vi "Tecella_FETAnalyser.vi"() -> ()   [LabVIEW 2009]
doc: "FET Analysis Code\n(C) Michael Walker 2014\nFree to re use and distribute for non commercial use. All rights reserved for commercial use.\nRed dsitrbution and modification must keep this license intact.\nSoftware is provided as is. The author accepts no responsibility for loss arising out of use of this program."
uses:
  TecellaChannel/TecellaChannel.lvclass
  <vilib>/measure/madcrms.llb/Basic Averaged DC-RMS for 1 Chan.vi
  TecellaClient/TecellaClient.lvclass
  <vilib>/measure/NI_MAPro.lvlib
panel:
  out "Running?":bool
  out "Igs nA":dbl format="%0.2e"
  in  "Channel 2":i8=2
  in  "Channel":i8
  out "Gate Resistance":dbl=-654868.3548789481 format="%#.4e"
  out "Gate IV":cluster{"Y":dbl[], "Y":dbl[]}[](graph)=[{"Y"=[90.50541857309688, 90.84377717312921, 91.26591980808492, 91.21758286507902, 91.67162788253441, 91.97325040553291], "Y"=[-1.1330458045852234e-05, -1.131434573173331e-05, -1.1781602836448501e-05, -1.2158630983030932e-05, -1.2596885922907083e-05, -1.1881499183117178e-05]}, {"Y"=[90.50541857309688, 90.84377717312921, 91.26591980808492, 91.21758286507902, 91.67162788253441, 91.97325040553291], "Y"=[-1.1358748353855137e-05, -1.1580328693617457e-05, -1.1856776546495164e-05, -1.1825122212149017e-05, -1.2122461925771009e-05, -1.2319984971201474e-05]}]
  in  "Recording?":bool
  in  "Dtitles":string[](array[string])
  in  "Clear Data":bool
  out "Data":cluster{"Y":dbl[], "Y":dbl[]}[](graph)
  out "Igs versus Vds":cluster{"Y":dbl[], "Y":dbl[]}[](graph)=[{"Y"=[90.50541857309688, 90.84377717312921, 91.26591980808492, 91.21758286507902, 91.67162788253441, 91.97325040553291], "Y"=[-1.1330458045852234e-05, -1.131434573173331e-05, -1.1781602836448501e-05, -1.2158630983030932e-05, -1.2596885922907083e-05, -1.1881499183117178e-05]}, {"Y"=[90.50541857309688, 90.84377717312921, 91.26591980808492, 91.21758286507902, 91.67162788253441, 91.97325040553291], "Y"=[-1.1358748353855137e-05, -1.1580328693617457e-05, -1.1856776546495164e-05, -1.1825122212149017e-05, -1.2122461925771009e-05, -1.2319984971201474e-05]}]
  out "Vgs FileNo":dbl
  out "Ids/Vds No":dbl
  out "File Path for saving":path=path "D:/Data/101116/101116_1/101116_1_FET0_100Hz_"
  in  "Details":string
  in  "Folder Path":path=path "D:/Data"
  out "File No":dbl
  out "Saving Data":bool
  out "File Name Out":path
  out "Vds Progress":u8(slide) scale=0.0..100.0
  out "Vgs Progress":u8(slide) scale=0.0..100.0
  in  "Start/Stop Recording":bool
  in  "Record All Data":bool
  in  "Vds Stabilisation":u32=700
  in  "Vgs Stabilisation":u32=600
  in  "clear":bool
  out "Channel Conducitivty (uS)":dbl format="%0.3e"
  out "Channel Resistance":dbl format="%#_3e"
  out "Live Channel Resistance":dbl format="%#_3e"
  out "Live channel Conductivity uS":dbl format="%#_3e"
  out "Vgs mV":dbl format="%0.2p"
  in  "Sample Freq Hz":dbl=100.0
  out "Vds mV":dbl format="%0.2p"
  in  "Set Vds mV":dbl
  in  "Set Vgs mV":dbl
  in  "stop":bool
  out "Ids nA":dbl format="%0.2e"
  in  "Samples to read":dbl=1024.0
  out "Measured Igs":dbl[][](graph)
  out "Masured Ids":dbl[][](graph)
  in  "Measure Channel Conductivity":bool
  in  "With Vds Sweep":bool
  in  "NoSteps":dbl=10.0
  in  "No steps":dbl=10.0
  in  "Vgs Min":dbl=-100.0
  in  "Vgs Max":dbl=100.0
  in  "Vds Min":dbl=-100.0
  in  "Vds Max":dbl=100.0
  in  "FET Analyse":bool
  out "S against Vds":cluster{"Y":dbl[], "Y":dbl[]}[](graph)
  out "Ids Agsint Vds":cluster{"Y":dbl[], "Y":dbl[]}[](graph)
  # "Note currents are recorded consecutivly and sample \nrate is incorrect"
  # "Drain Source Voltage Sweep"
  # "Gate Source Voltage Sweep"
  # "NB new file created each time recording is started"
  # "Controls actual recording"
  # "Used to indicate if the current file has been recorded into"
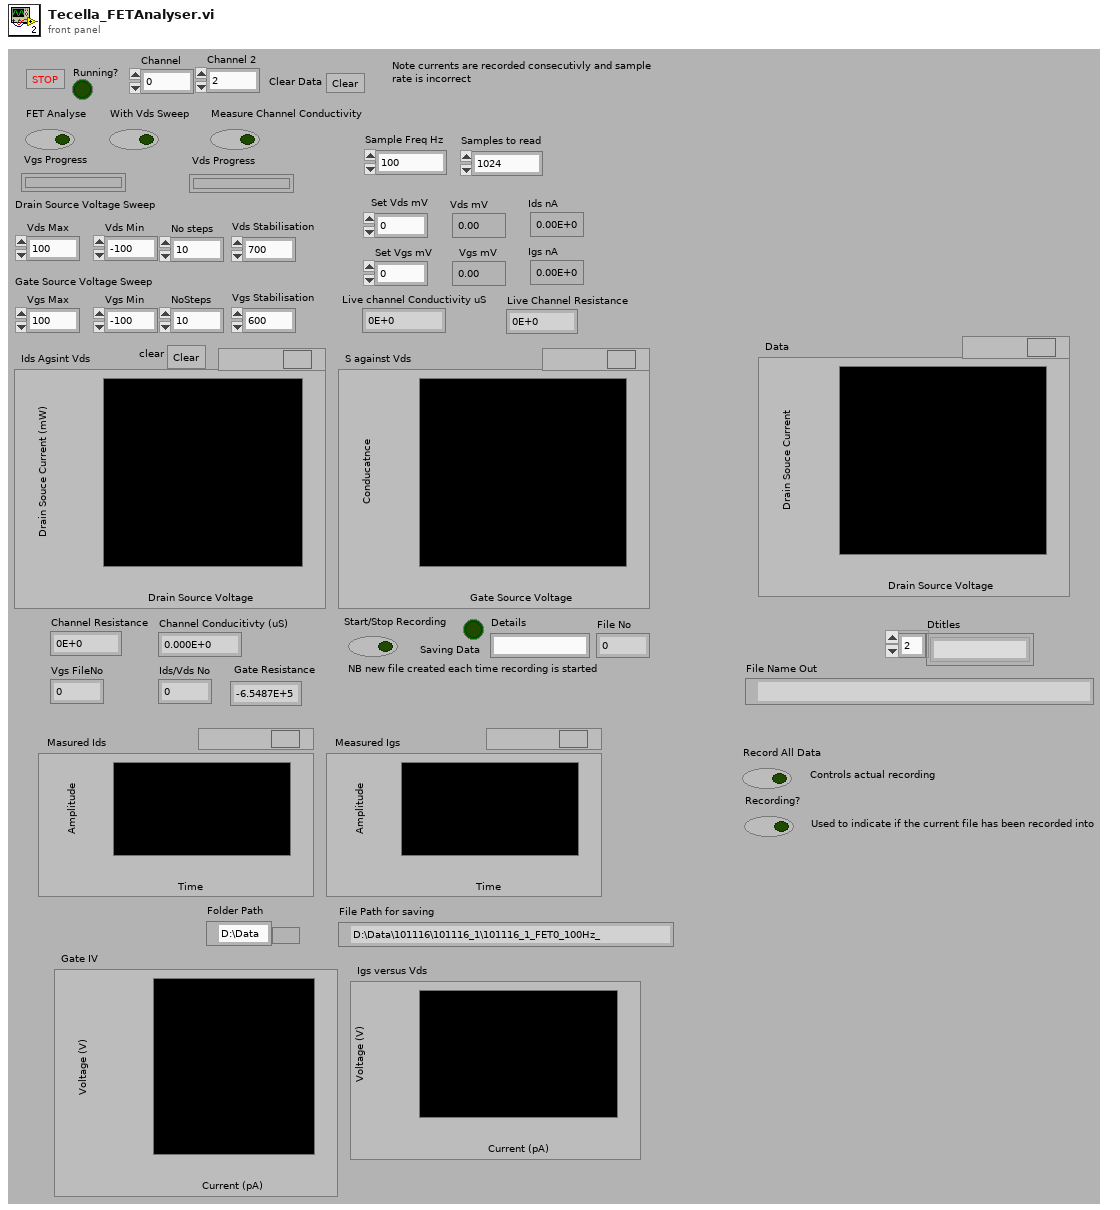
[diagram p1: front panel]
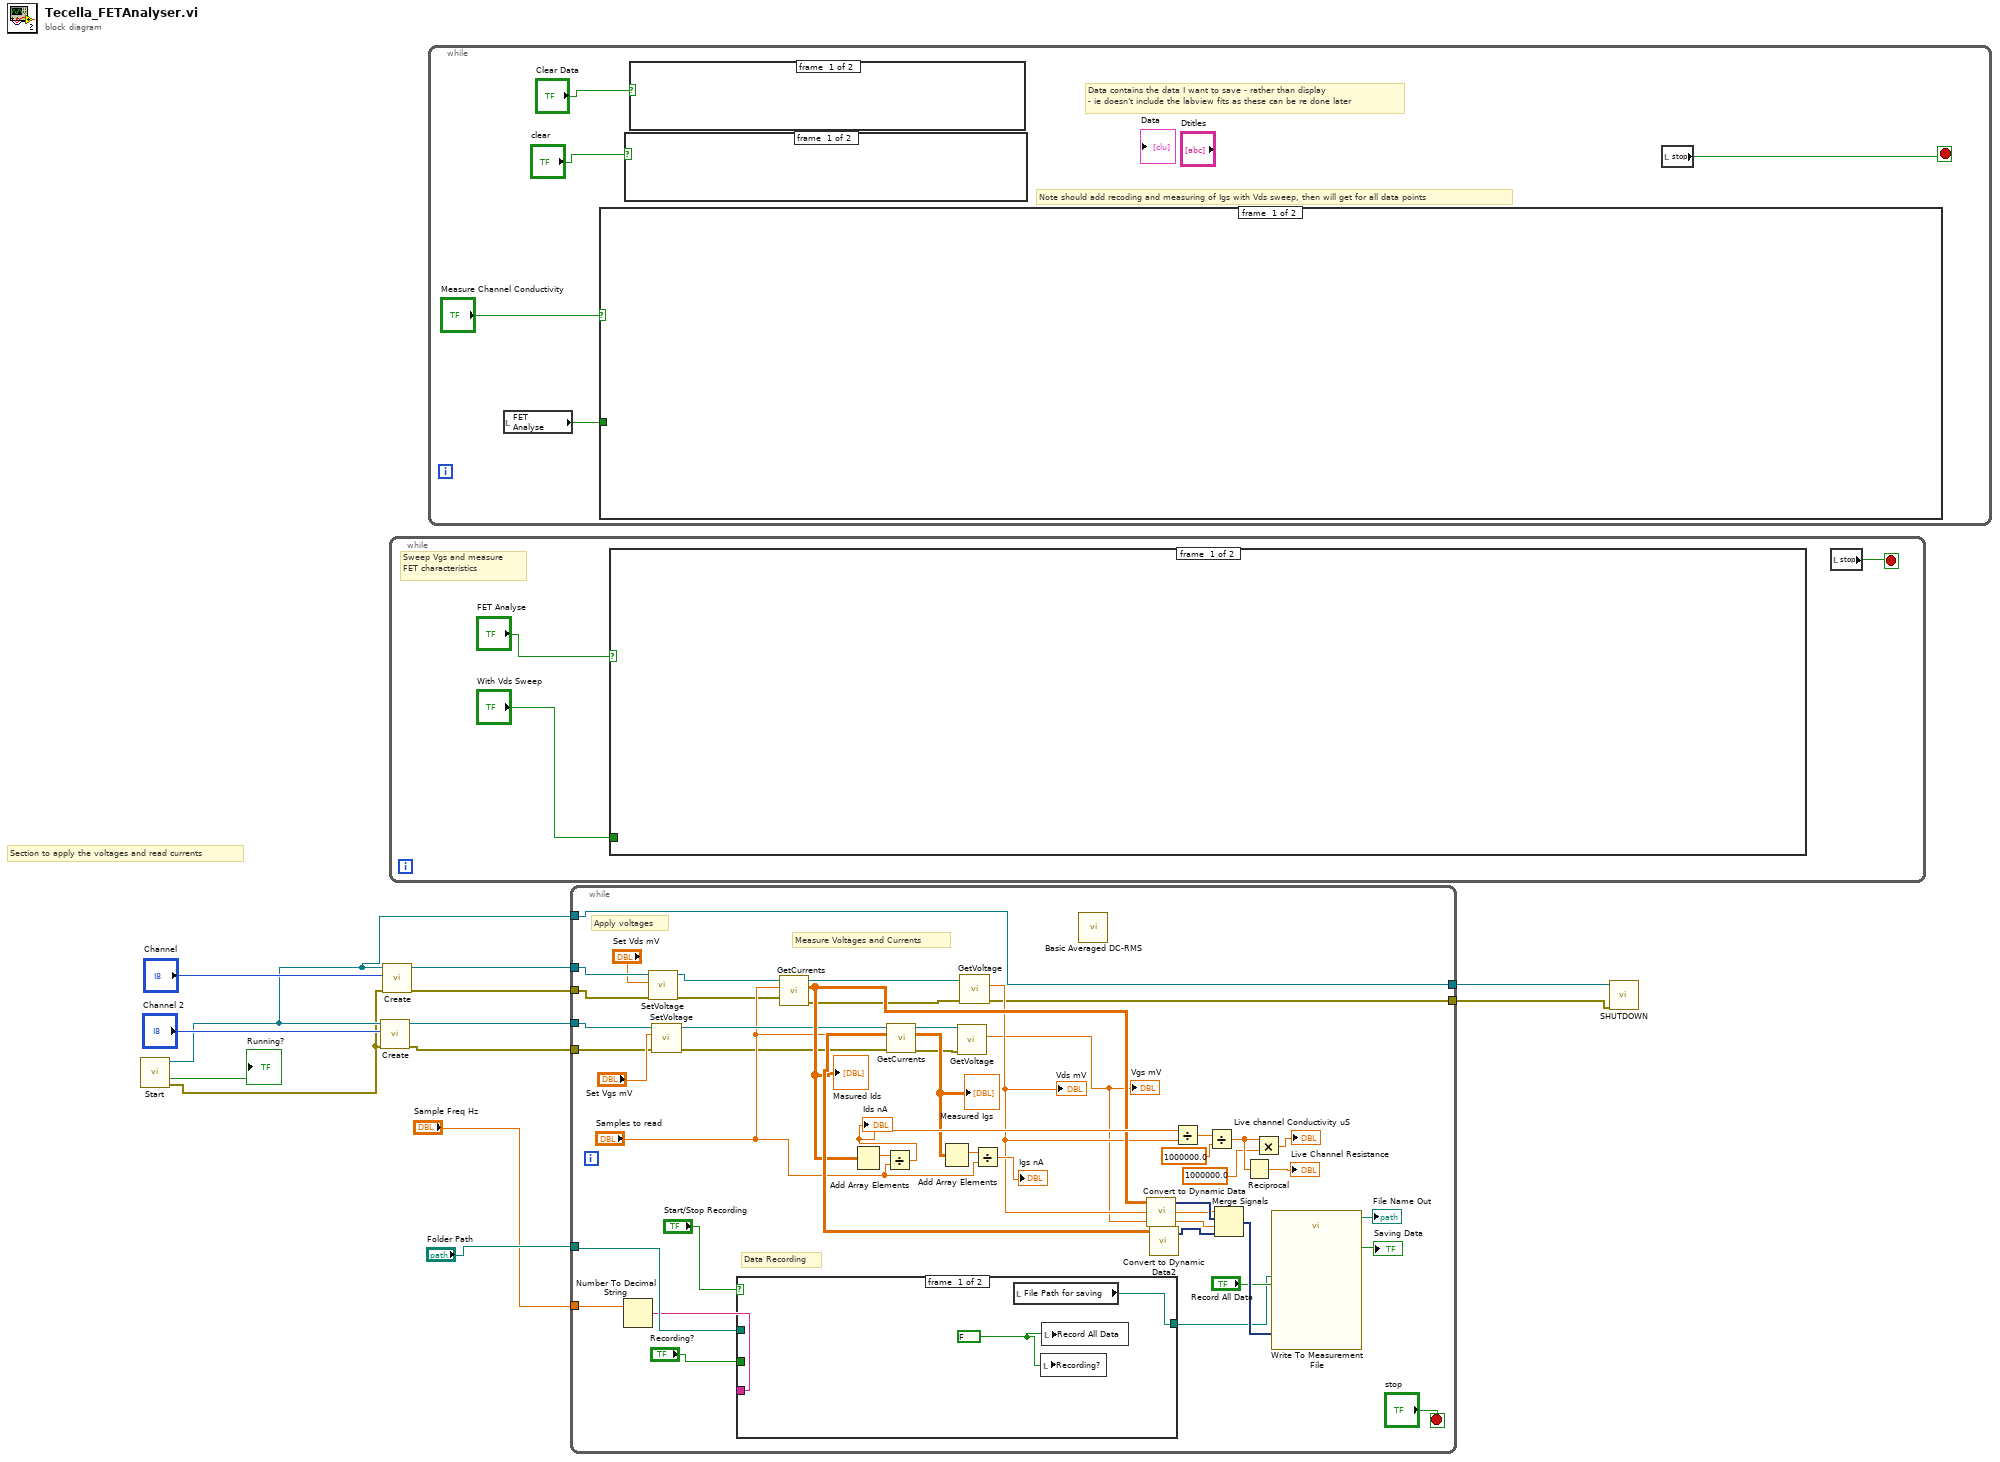
[diagram p0: block diagram]
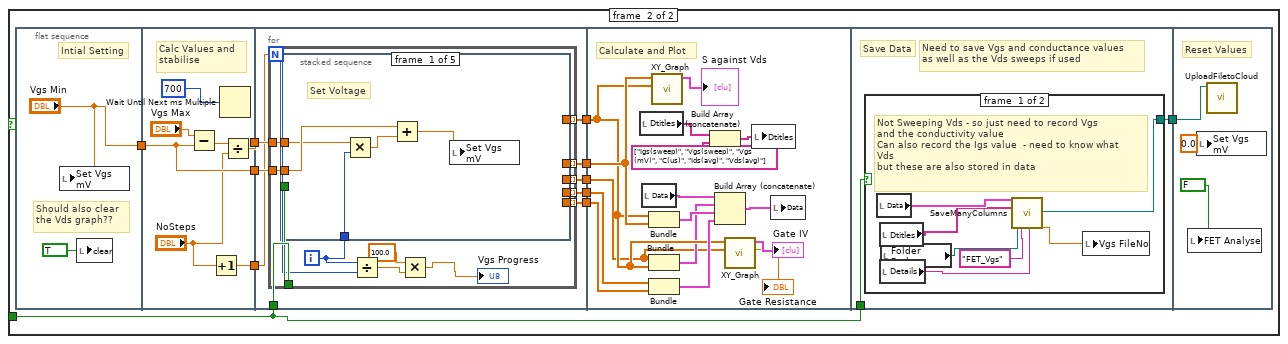
[diagram p2: hidden frame]
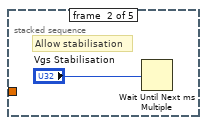
[diagram p3: hidden frame]
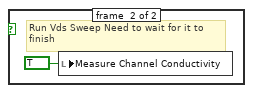
[diagram p5: hidden frame]
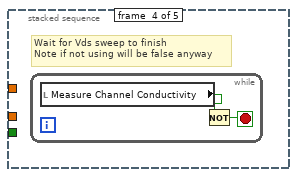
[diagram p6: hidden frame]
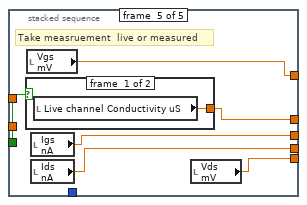
[diagram p7: hidden frame]
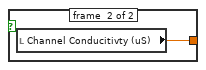
[diagram p8: hidden frame]
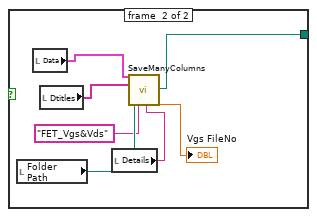
[diagram p9: hidden frame]
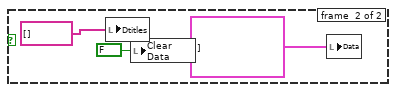
[diagram p10: hidden frame]
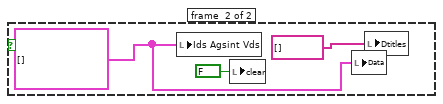
[diagram p11: hidden frame]
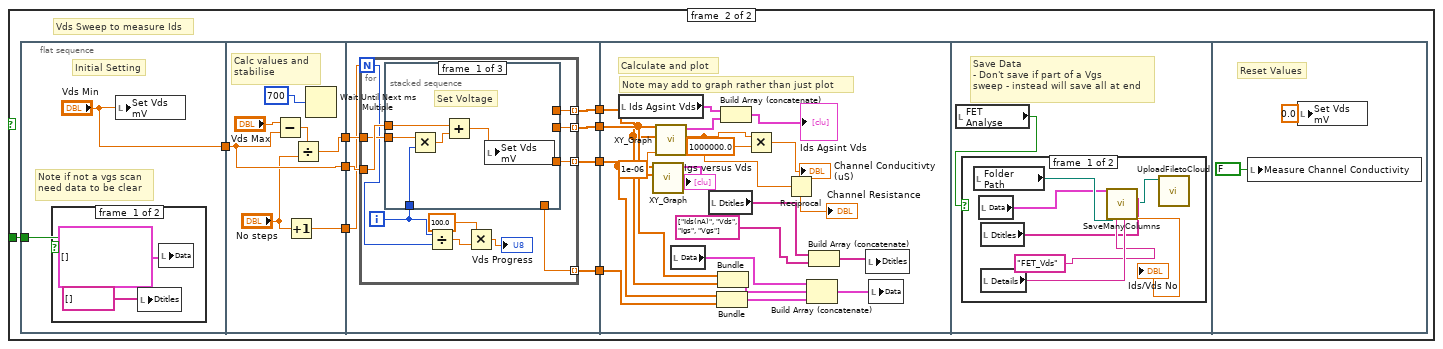
[diagram p12: hidden frame]
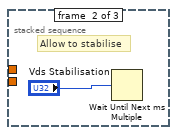
[diagram p14: hidden frame]
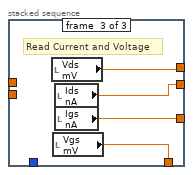
[diagram p15: hidden frame]
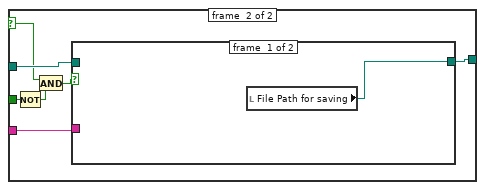
[diagram p17: hidden frame]
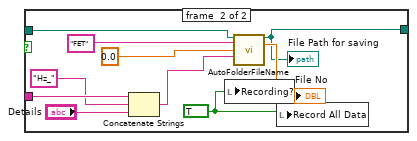
[diagram p18: hidden frame]
diagram:
  # "Section to apply the voltages and read currents"
  n1 = call "Start.vi"() -> ("TecellaClient"=w6:refnum<class "TecellaClient.lvclass">, "Running?"=→"Running?":bool, "error out"=w1:errorcluster)  [unwired: 11 in, 2 out]
  n2 = call "Create.vi"("error in (no error)"=w1, "Channel"="Channel 2", "TecellaClient.lvclass"=w6) -> ("error out"=w2:errorcluster, "TecellaChannel out"=w7:refnum<class "TecellaChannel.lvclass">)  [unwired: 7 in]
  n3 = call "Create.vi"("error in (no error)"=w1, "Channel"="Channel", "TecellaClient.lvclass"=w6) -> ("error out"=w3:errorcluster, "TecellaChannel out"=w8:refnum<class "TecellaChannel.lvclass">)  [unwired: 7 in]
  n4 = while {
    stop <- w14 stop-if-true
    # "Sweep Vgs and measure \nFET characteristics"
    n5 = case shown="True" "FET Analyse" {
      tunnel: "With Vds Sweep" -> [_ w22]
      frame #0 {
      }
      frame #1 {
        n6 = flat-sequence {
          tunnel: ["Vgs Min"] -> w27
          tunnel: w27 -> [w33]
          tunnel: [w33] -> w24
          tunnel: [w32] -> w23
          tunnel: [w30] -> w18
          tunnel: w22 -> [w45]
          tunnel: [w44] -> w26
          tunnel: [w43] -> w25
          tunnel: w24 -> [w42]
          tunnel: w23 -> [w41]
          tunnel: [w40] -> w21
          tunnel: [w39] -> w20
          tunnel: [w38] -> w19
          tunnel: w18 -> [w37]
          tunnel: w26 -> [w80]
          tunnel: w25 -> [w87]
          tunnel: w21 -> [w77]
          tunnel: w20 -> [w85]
          tunnel: w19 -> [w86]
          tunnel: w22 -> [w94]
          tunnel: [w93] -> w17
          tunnel: w17 -> [w109]
          frame #0 {
            # "Should also clear \nthe Vds graph??"
            # "Intial Setting"
            n7 = local write "Set Vgs mV"("Vgs Min") -> ()
            n8 = local write "clear"(TRUE ("clear")) -> ()
          }
          frame #1 {
            # "Calc Values and \nstabilise"
            n9 = Subtract(x="Vgs Max", y=w33) -> (x-y=w36:dbl)
            n10 = Increment(x="NoSteps") -> (x+1=w30:dbl)
            n11 = Wait Until Next ms Multiple(millisecond multiple=u32 700) -> ()  [unwired: 1 out]
            n12 = Divide(x=w36, y="NoSteps") -> (x/y=w32:dbl)
          }
          frame #2 {
            n13 = for {
              N: w37 -> [w53]
              tunnel: w45 -> [w58]
              tunnel: [w57] -> w44 mode=indexing
              tunnel: [w56] -> w43 mode=indexing
              tunnel: w42 -> [w55]
              tunnel: w41 -> [w52]
              tunnel: [w48] -> w40 mode=indexing
              tunnel: [w47] -> w39 mode=indexing
              tunnel: [w46] -> w38 mode=indexing
              i -> [w54]
              n14 = stacked-sequence {
                tunnel: w58 -> [_ _ w65 _ w74]
                tunnel: [_ _ _ _ w73] -> w57
                tunnel: [_ _ _ _ w72] -> w56
                tunnel: w54 -> [w63 _ _ _ _]
                tunnel: w55 -> [w61 _ _ _ _]
                tunnel: w52 -> [w59 _ _ _ _]
                tunnel: [_ _ _ _ w69] -> w48
                tunnel: [_ _ _ _ w71] -> w47
                tunnel: [_ _ _ _ w70] -> w46
                frame #0 {
                  # "Set Voltage"
                  n15 = Multiply(x=w59, y=w63) -> (x*y=w62:dbl)
                  n16 = Add(x=w61, y=w62) -> (x+y=w60:dbl)
                  n17 = local write "Set Vgs mV"(w60) -> ()
                }
                frame #1 {
                  # "Allow stabilisation"
                  n18 = Wait Until Next ms Multiple(millisecond multiple="Vgs Stabilisation") -> ()  [unwired: 1 out]
                }
                frame #2 {
                  # "Now run Vds sweep and wait for it to finish\nOr just take the live values"
                  n19 = case shown="True" w65 {
                    frame #0 {
                      # "Just take the live values"
                    }
                    frame #1 {
                      # "Run Vds Sweep Need to wait for it to \nfinish"
                      n20 = local write "Measure Channel Conductivity"(TRUE ("Measure Channel Conductivity")) -> ()
                    }
                  }
                }
                frame #3 {
                  # "Wait for Vds sweep to finish\nNote if not using will be false anyway"
                  n21 = while {
                    stop <- w68 stop-if-true
                    n22 = local read "Measure Channel Conductivity"() -> (w67:bool)
                    n23 = Not(x=w67) -> (.not. x?=w68:bool)
                  }
                }
                frame #4 {
                  # "Take measruement  live or measured"
                  n24 = case shown="True" w74 {
                    tunnel: [w75 w76] -> w72
                    frame #0 {
                      n25 = local read "Live channel Conductivity uS"() -> (w75:dbl)
                    }
                    frame #1 {
                      n26 = local read "Channel Conducitivty (uS)"() -> (w76:dbl)
                    }
                  }
                  n27 = local read "Vgs mV"() -> (w73:dbl)
                  n28 = local read "Igs nA"() -> (w69:dbl)
                  n29 = local read "Ids nA"() -> (w70:dbl)
                  n30 = local read "Vds mV"() -> (w71:dbl)
                }
              }
              n31 = Divide(x=w54, y=w53) -> (x/y=w50:dbl)
              n32 = Multiply(x=100.0, y=w50) -> (x*y=→"Vgs Progress":dbl)
            }
          }
          frame #3 {
            # "Calculate and Plot"
            n33 = local read "Dtitles"() -> (w90:string[])
            n34 = local read "Data"() -> (w79:cluster{"Y":dbl[], "Y":dbl[]}[])
            n35 = Bundle(w80, w87) -> (w81:cluster{dbl[], dbl[]})  [unwired: 1 out]
            n36 = Bundle(w77, w80) -> (w78:cluster{dbl[], dbl[]})  [unwired: 1 out]
            n37 = Bundle(w86, w85) -> (w82:cluster{dbl[], dbl[]})  [unwired: 1 out]
            n38 = call "XY_Graph.vi"("X"=w80, "Y"=w87) -> ("I-V Curve"=→"S against Vds":cluster{"Y":dbl[], "Y":dbl[]}[])  [unwired: 8 in, 1 out]
            n39 = Build Array (concatenate)(w90, string[] ["Igs(sweep)", "Vgs(sweep)", "Vgs (mV)", "C(us)", "Ids(avg)", "Vds(avg)"] ("ColumnTitle Array")) -> (w89:string[])
            n40 = Build Array (concatenate)(w79, w78, w81, w82) -> (w91:cluster{"Y":dbl[], "Y":dbl[]}[])
            n41 = call "XY_Graph.vi"("X"=w77, "Y"=w80) -> ("Gradient"=→"Gate Resistance":dbl, "I-V Curve"=→"Gate IV":cluster{"Y":dbl[], "Y":dbl[]}[])  [unwired: 8 in]
            n42 = local write "Dtitles"(w89) -> ()
            n43 = local write "Data"(w91) -> ()
          }
          frame #4 {
            # "Need to save Vgs and conductance values\nas well as the Vds sweeps if used"
            # "Save Data"
            n44 = case shown="False" w94 {
              tunnel: [w95 w102] -> w93
              frame #0 {
                # "Not Sweeping Vds - so just need to record Vgs\nand the conductivity value \nCan also record the Igs value  - need to know what \nVds\nbut these are also stored in data"
                n45 = local read "Data"() -> (w100:cluster{"Y":dbl[], "Y":dbl[]}[])
                n46 = local read "Dtitles"() -> (w96:string[])
                n47 = local read "Details"() -> (w97:string)
                n48 = local read "Folder Path"() -> (w101:path)
                n49 = call "SaveManyColumns.vi"("InputCluster"=w100, "ColumnTitle Array"=w96, "Folder Path"=w101, "Capillary Type"="FET_Vgs" ("Comments"), "Details"=w97) -> ("Saved Path"=w95:path, "File No"=w99:dbl)  [unwired: 20 in, 1 out]
                n50 = local write "Vgs FileNo"(w99) -> ()
              }
              frame #1 {
                n51 = local read "Folder Path"() -> (w107:path)
                n52 = local read "Data"() -> (w104:cluster{"Y":dbl[], "Y":dbl[]}[])
                n53 = local read "Dtitles"() -> (w103:string[])
                n54 = local read "Details"() -> (w105:string)
                n55 = call "SaveManyColumns.vi"("InputCluster"=w104, "ColumnTitle Array"=w103, "Folder Path"=w107, "Capillary Type"="FET_Vgs&Vds" ("Comments"), "Details"=w105) -> ("Saved Path"=w102:path, "File No"=→"Vgs FileNo":dbl)  [unwired: 20 in, 1 out]
              }
            }
          }
          frame #5 {
            # "Reset Values"
            n56 = local write "FET Analyse"(FALSE ("FET Analyse")) -> ()
            n57 = local write "Set Vgs mV"(0.0 ("Set Vgs")) -> ()
            n58 = call "UploadFiletoCloud.vi"("File  To Upload"=w109) -> ()  [unwired: 8 in, 3 out]
          }
        }
      }
    }
    n59 = local read "stop"() -> (w14:bool)
  }
  n60 = while {
    stop <- w114 stop-if-true
    # "Data contains the data I want to save - rather than display \n- ie doesn't include the labview fits as these can be re done later"
    # "Note should add recoding and measuring of Igs with Vds sweep, then will get for all data points"
    n61 = local read "FET Analyse"() -> (w112:bool)
    n62 = case shown="True" "Measure Channel Conductivity" {
      tunnel: w112 -> [_ w124]
      frame #0 {
      }
      frame #1 {
        # "Vds Sweep to measure Ids"
        n63 = flat-sequence {
          tunnel: ["Vds Min"] -> w129
          tunnel: w124 -> [w132]
          tunnel: [w139] -> w131
          tunnel: [w140] -> w130
          tunnel: w129 -> [w139]
          tunnel: [w136] -> w123
          tunnel: w131 -> [w149]
          tunnel: w130 -> [w148]
          tunnel: [w147] -> w128
          tunnel: [w146] -> w127
          tunnel: [w145] -> w126
          tunnel: [w144] -> w125
          tunnel: w123 -> [w143]
          tunnel: w128 -> [w181]
          tunnel: w127 -> [w182]
          tunnel: w126 -> [w172]
          tunnel: w125 -> [w174]
          frame #0 {
            # "Note if not a vgs scan\nneed data to be clear"
            # "Initial Setting"
            n64 = case shown="False" w132 {
              frame #0 {
                n65 = local write "Dtitles"(string[] [] ("ColumnTitle Array")) -> ()
                n66 = local write "Data"(cluster{"Y":dbl[], "Y":dbl[]}[] [] ("Ids Agsint Vds")) -> ()
              }
              frame #1 {
                # "leave data as collecting"
              }
            }
            n67 = local write "Set Vds mV"("Vds Min") -> ()
          }
          frame #1 {
            # "Calc values and \nstabilise"
            n68 = Subtract(x="Vds Max", y=w139) -> (x-y=w141:dbl)
            n69 = Increment(x="No steps") -> (x+1=w136:dbl)
            n70 = Divide(x=w141, y="No steps") -> (x/y=w140:dbl)
            n71 = Wait Until Next ms Multiple(millisecond multiple=u32 700) -> ()  [unwired: 1 out]
          }
          frame #2 {
            n72 = for {
              N: w143 -> [w155]
              tunnel: w149 -> [w160]
              tunnel: w148 -> [w159]
              tunnel: [w158] -> w147 mode=indexing
              tunnel: [w157] -> w146 mode=indexing
              tunnel: [w151] -> w145 mode=indexing
              tunnel: [w150] -> w144 mode=indexing
              i -> [w156]
              n73 = stacked-sequence {
                tunnel: w160 -> [w165 _ _]
                tunnel: w156 -> [w161 _ _]
                tunnel: w159 -> [w163 _ _]
                tunnel: [_ _ w169] -> w158
                tunnel: [_ _ w170] -> w157
                tunnel: [_ _ w168] -> w151
                tunnel: [_ _ w167] -> w150
                frame #0 {
                  # "Set Voltage"
                  n74 = Multiply(x=w163, y=w161) -> (x*y=w164:dbl)
                  n75 = Add(x=w165, y=w164) -> (x+y=w162:dbl)
                  n76 = local write "Set Vds mV"(w162) -> ()
                }
                frame #1 {
                  # "Allow to stabilise"
                  n77 = Wait Until Next ms Multiple(millisecond multiple="Vds Stabilisation") -> ()  [unwired: 1 out]
                }
                frame #2 {
                  # "Read Current and Voltage"
                  n78 = local read "Vds mV"() -> (w169:dbl)
                  n79 = local read "Vgs mV"() -> (w167:dbl)
                  n80 = local read "Ids nA"() -> (w170:dbl)
                  n81 = local read "Igs nA"() -> (w168:dbl)
                }
              }
              n82 = Divide(x=w156, y=w155) -> (x/y=w154:dbl)
              n83 = Multiply(x=100.0, y=w154) -> (x*y=→"Vds Progress":dbl)
            }
          }
          frame #3 {
            # "Note may add to graph rather than just plot"
            # "Calculate and plot"
            n84 = local read "Ids Agsint Vds"() -> (w188:cluster{"Y":dbl[], "Y":dbl[]}[])
            n85 = call "XY_Graph.vi"("X"=w181, "Y"=w172) -> ("I-V Curve"=→"Igs versus Vds":cluster{"Y":dbl[], "Y":dbl[]}[])  [unwired: 8 in, 1 out]
            n86 = call "XY_Graph.vi"("Scaling of Gradient"=1e-06, "X"=w181, "Y"=w182) -> ("Gradient"=w173:dbl, "I-V Curve"=w189:cluster{"Y":dbl[], "Y":dbl[]}[])  [unwired: 7 in]
            n87 = local read "Data"() -> (w184:cluster{"Y":dbl[], "Y":dbl[]}[])
            n88 = local read "Dtitles"() -> (w177:string[])
            n89 = Bundle(w172, w174) -> (w171:cluster{dbl[], dbl[]})  [unwired: 1 out]
            n90 = Bundle(w182, w181) -> (w185:cluster{dbl[], dbl[]})  [unwired: 1 out]
            n91 = Build Array (concatenate)(w188, w189) -> (→"Ids Agsint Vds":cluster{"Y":dbl[], "Y":dbl[]}[])
            n92 = Multiply(x=w173, y=1000000.0) -> (x*y=→"Channel Conducitivty (uS)":dbl)
            n93 = Reciprocal(x=w173) -> (1/x=→"Channel Resistance":dbl)
            n94 = Build Array (concatenate)(w184, w185, w171) -> (w186:cluster{"Y":dbl[], "Y":dbl[]}[])
            n95 = Build Array (concatenate)(w177, string[] ["Ids(nA)", "Vds", "Igs", "Vgs"] ("ColumnTitle Array")) -> (w183:string[])
            n96 = local write "Dtitles"(w183) -> ()
            n97 = local write "Data"(w186) -> ()
          }
          frame #4 {
            # "Save Data\n- Don't save if part of a Vgs\nsweep - instead will save all at end"
            n98 = local read "FET Analyse"() -> (w191:bool)
            n99 = case shown="False" w191 {
              frame #0 {
                n100 = local read "Folder Path"() -> (w197:path)
                n101 = local read "Data"() -> (w194:cluster{"Y":dbl[], "Y":dbl[]}[])
                n102 = local read "Dtitles"() -> (w193:string[])
                n103 = local read "Details"() -> (w198:string)
                n104 = call "SaveManyColumns.vi"("InputCluster"=w194, "ColumnTitle Array"=w193, "Folder Path"=w197, "Capillary Type"="FET_Vds" ("Comments"), "Details"=w198) -> ("Saved Path"=w192:path, "File No"=→"Ids/Vds No":dbl)  [unwired: 20 in, 1 out]
                n105 = call "UploadFiletoCloud.vi"("File  To Upload"=w192) -> ()  [unwired: 8 in, 3 out]
              }
              frame #1 {
                # "If part of the Vgs \nsweep don't save \nindividual files"
              }
            }
          }
          frame #5 {
            # "Reset Values"
            n106 = local write "Measure Channel Conductivity"(FALSE ("Measure Channel Conductivity")) -> ()
            n107 = local write "Set Vds mV"(0.0 ("Set Vds")) -> ()
          }
        }
      }
    }
    n108 = case shown="True" "clear" {
      frame #0 {
      }
      frame #1 {
        w121 = cluster{"Y":dbl[], "Y":dbl[]}[] [] ("Ids Agsint Vds")
        n109 = local write "Ids Agsint Vds"(w121) -> ()
        n110 = local write "clear"(FALSE ("clear")) -> ()
        n111 = local write "Data"(w121) -> ()
        n112 = local write "Dtitles"(string[] [] ("ColumnTitle Array")) -> ()
      }
    }
    n113 = case shown="True" "Clear Data" {
      frame #0 {
      }
      frame #1 {
        n114 = local write "Dtitles"(string[] [] ("ColumnTitle Array")) -> ()
        n115 = local write "Clear Data"(FALSE ("Clear Data")) -> ()
        n116 = local write "Data"(cluster{"Y":dbl[], "Y":dbl[]}[] [] ("Ids Agsint Vds")) -> ()
      }
    }
    n117 = local read "stop"() -> (w114:bool)
  }
  n118 = while {
    tunnel: "Folder Path" -> [w237]
    tunnel: "Sample Freq Hz" -> [w222]
    tunnel: w8 -> [w219]
    tunnel: w7 -> [w217]
    tunnel: w6 -> [w210]
    tunnel: [w210] -> w5
    tunnel: [w209] -> w4
    tunnel: w3 -> [w206]
    tunnel: w2 -> [w203]
    stop <- "stop" stop-if-true
    # "Data Recording"
    # "Apply voltages"
    # "Measure Voltages and Currents"
    n119 = Number To Decimal String(number=w222) -> (decimal integer string=w236:string)  [unwired: 1 in]
    n120 = call-dynamic "SetVoltage.vi"("error in (no error)"=w206, "Voltage"="Set Vds mV", "TecellaChannel in"=w219) -> ("error out"=w207:errorcluster, "TecellaChannel out"=w218:refnum<class "TecellaChannel.lvclass">)  [unwired: 7 in]
    n121 = call-dynamic "SetVoltage.vi"("error in (no error)"=w203, "Voltage"="Set Vgs mV", "TecellaChannel in"=w217) -> ("error out"=w204:errorcluster, "TecellaChannel out"=w216:refnum<class "TecellaChannel.lvclass">)  [unwired: 7 in]
    n122 = case shown="True" "Start/Stop Recording" {
      selector: "Start/Stop Recording" -> [_ w247]
      tunnel: [w245 w253] -> w238
      tunnel: w237 -> [_ w252]
      tunnel: w236 -> [_ w251]
      tunnel: "Recording?" -> [_ w250]
      frame #0 {
        w246 = FALSE ("Record All Data")
        n123 = local read "File Path for saving"() -> (w245:path)
        n124 = local write "Recording?"(w246) -> ()
        n125 = local write "Record All Data"(w246) -> ()
      }
      frame #1 {
        n126 = Not(x=w250) -> (.not. x?=w249:bool)
        n127 = And(x=w247, y=w249) -> (x .and. y?=w248:bool)
        n128 = case shown="True" w248 {
          tunnel: [w254 w263] -> w253
          tunnel: w252 -> [_ w262]
          tunnel: w251 -> [_ w258]
          frame #0 {
            n129 = local read "File Path for saving"() -> (w254:path)
          }
          frame #1 {
            w255 = TRUE ("New File")
            n130 = Concatenate Strings(w258, "Hz_" ("element"), "Details") -> (w259:string)
            n131 = local write "Recording?"(w255) -> ()
            n132 = call "AutoFolderFileName.vi"("Folder Path"=w262, "Capillary Type"="FET" ("Details"), "Capilary"=0.0, "Details"=w259) -> ("File Path for saving"=w263:path, "File No"=→"File No":dbl)  [unwired: 5 in, 5 out]
            "File Path for saving" <- w263
            n133 = local write "Record All Data"(w255) -> ()
          }
        }
      }
    }
    n134 = call-dynamic "GetCurrents.vi"("error in (no error)"=w207, "Samples"="Samples to read", "TecellaChannel in"=w218) -> ("error out"=w208:errorcluster, "Currents (nA)"=w220:dbl[][], "TecellaChannel out"=w201:refnum<class "TecellaChannel.lvclass">)  [unwired: 6 in]
    "Masured Ids" <- w220
    n135 = Add Array Elements(numeric array=w220) -> (sum=w226:dbl)
    n136 = Divide(x=w226, y="Samples to read") -> (x/y=w225:dbl)
    "Ids nA" <- w225
    n137 = call-dynamic "GetCurrents.vi"("error in (no error)"=w204, "Samples"="Samples to read", "TecellaChannel in"=w216) -> ("error out"=w205:errorcluster, "Currents (nA)"=w221:dbl[][], "TecellaChannel out"=w202:refnum<class "TecellaChannel.lvclass">)  [unwired: 6 in]
    "Measured Igs" <- w221
    n138 = Add Array Elements(numeric array=w221) -> (sum=w223:dbl)
    n139 = call-dynamic "GetVoltage.vi"("error in (no error)"=w205, "TecellaChannel in"=w202) -> ("Voltage (mV)"=w211:dbl)  [unwired: 7 in, 2 out]
    "Vgs mV" <- w211
    n140 = call-dynamic "GetVoltage.vi"("error in (no error)"=w208, "TecellaChannel in"=w201) -> ("error out"=w209:errorcluster, "Voltage (mV)"=w212:dbl)  [unwired: 7 in, 1 out]
    "Vds mV" <- w212
    n141 = Divide(x=w223, y="Samples to read") -> (x/y=→"Igs nA":dbl)
    n142 = call-poly <vilib>:"Basic Averaged DC-RMS.vi"() -> ()  [unwired: 5 in, 7 out]
    n143 = call "Convert to Dynamic Data"("2D Array"=w220) -> ("Dynamic Data Type"=w227:dynamicdata)  [unwired: 3 in]
    n144 = call "Convert to Dynamic Data2"("2D Array"=w221) -> ("Dynamic Data Type"=w228:dynamicdata)  [unwired: 3 in]
    n145 = Divide(x=w225, y=w212) -> (x/y=w235:dbl)
    n146 = Divide(x=w235, y=1000000.0) -> (x/y=w232:dbl)
    n147 = Merge Signals(w212, w227, w211, w228) -> (w242:dynamicdata)
    n148 = Reciprocal(x=w232) -> (1/x=→"Live Channel Resistance":dbl)
    n149 = Multiply(x=w232, y=1000000.0) -> (x*y=→"Live channel Conductivity uS":dbl)
    n150 = call "Write To Measurement File"("Signals"=w242, "Enable"="Record All Data", "Filename"=w238) -> ("Filename Out"=→"File Name Out":path, "Saving Data"=→"Saving Data":bool)  [unwired: 14 in, 1 out]
  }
  n151 = call-dynamic "SHUTDOWN.vi"("error in (no error)"=w4, "TecellaClient in"=w5) -> ()  [unwired: 8 in, 2 out]
